vi "CheckForNewTopic.vi"(3 "ROS":T1) -> (1 "new?":bool)   [LabVIEW 2012]
uses:
  <userlib>/ROSforLV/ROS/Code/SubVIs/_ROSControl.ctl
  <userlib>/ROSforLV/ROS/Code/SubVIs/_ROSDirection.ctl
  <userlib>/ROSforLV/ROS/Code/_ROSDefinition.vi
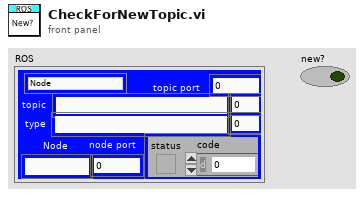
[diagram p1: front panel]
types:
  T1 = typedef "_ROSControl.ctl" = cluster{"topic port":u16, "Node":string, "topic":string, "type":string, "node port":u16, "error ":errorcluster, "Direction":T2, "Update (ms)":u16, "queue size":u16}
  T2 = typedef "_ROSDirection.ctl" = enum16{"Node", "Publisher", "Subscriber", "Service Client"}
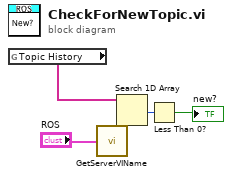
[diagram p0: block diagram]
diagram:
  n1 = global read "_ROSDefinition.vi" "Topic History"() -> (w4:string[])
  n2 = call <userlib>:"GetServerVIName.vi"("ROS"="ROS") -> ("vi name"=w5:string)
  n3 = Search 1D Array(1D array=w4, element=w5) -> (index of element=w3:i32)  [unwired: 1 in]
  n4 = Less Than 0?(x=w3) -> (x < 0?=→"new?":bool)
